vi "ZLIB Store__ogtk.vi"   [LabVIEW 2014, in "ZLIB.lvlib"]
uses:
  ZLIB.lvlib
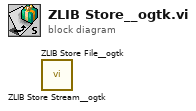
[diagram p0: block diagram]
diagram:
  n1 = call "ZLIB Store Stream__ogtk.vi"() -> ()  [unwired: 10 in, 2 out]
  n2 = call "ZLIB Store File__ogtk.vi"() -> ()  [unwired: 10 in, 2 out]
